vi "IMU model SUBVI.vi"(11 "Enum 3":enum16{"None", "Disc", "Box", "STL"}(ring)=enum."Disc") -> (3 "SceneObject out":refnum<vi>)   [LabVIEW 2021, in "IMU Display.lvlib"]
uses:
  <vilib>/picture/3D Picture Control/Object/Create Object (name).vi
  <vilib>/picture/3D Picture Control/Object/Create Object (drawable).vi
  <vilib>/picture/3D Picture Control/Object/Add Object (no reference).vi
  IMU Display.lvlib
  <vilib>/picture/3D Picture Control/NI_3D Picture Control.lvlib
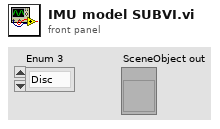
[diagram p1: front panel]
types:
  T1 = cluster{"Red":sgl, "Green":sgl, "Blue":sgl, "Alpha":sgl}
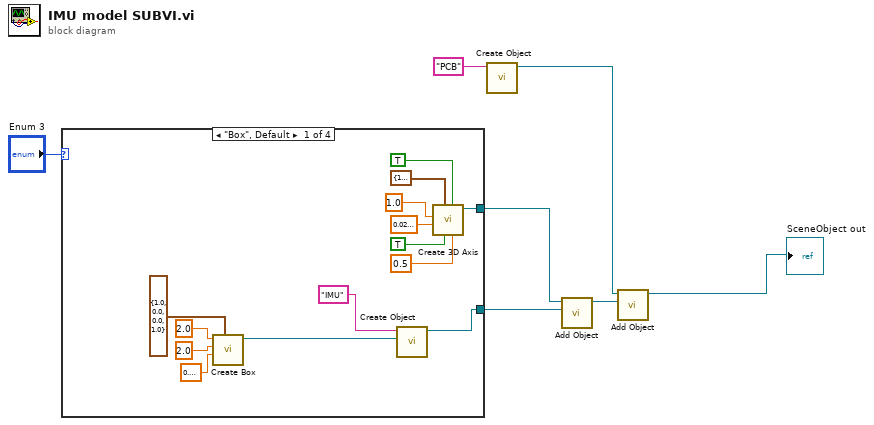
[diagram p0: block diagram]
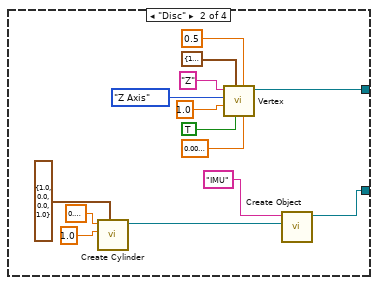
[diagram p2: hidden frame]
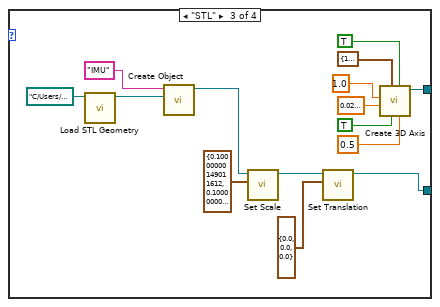
[diagram p3: hidden frame]
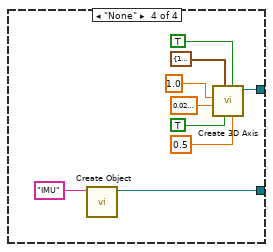
[diagram p4: hidden frame]
diagram:
  n1 = case shown="\"Box\", Default" "Enum 3" {
    tunnel: [w16 w32 w43 w58] -> w2
    tunnel: [w8 w23 w36 w51] -> w4
    frame "Box", Default {
      n2 = call <vilib>:"Create Box.vi"("Color"=T1 {"Red"=1.0, "Green"=0.0, "Blue"=0.0, "Alpha"=1.0}, "Length Z"=sgl 0.2, "Length Y"=sgl 2.0, "Length X"=sgl 2.0) -> ("New Box Refnum"=w17:refnum<vi>)  [unwired: 6 in, 1 out]
      n3 = call-poly <vilib>:"Create Object.vi"("Geometry"=w17, "Name"="IMU") -> ("Scene:New Object"=w16:refnum<vi>)  [unwired: 8 in, 1 out]
      n4 = call <vilib>:"Create 3D Axis.vi"("Character Size"=sgl 0.5, "Half plane?"=TRUE, "Axis label?"=TRUE, "Color"=T1 {"Red"=1.0, "Green"=0.0, "Blue"=0.0, "Alpha"=1.0}, "Radius"=sgl 0.03, "Length"=sgl 1.0) -> ("New Object Refnum"=w8:refnum<vi>)  [unwired: 4 in, 1 out]
    }
    frame "Disc" {
      n5 = call <vilib>:"Create Cylinder.vi"("Color"=T1 {"Red"=1.0, "Green"=0.0, "Blue"=0.0, "Alpha"=1.0}, "Radius"=sgl 1.0 ("Length Y"), "Height"=sgl 0.2 ("Length Z")) -> ("New Cylinder Refnum"=w33:refnum<vi>)  [unwired: 7 in, 1 out]
      n6 = call "Vertex.vi"("Radius"=sgl 0.01, "Font Size"=sgl 0.5 ("Character Size"), "Vertex label?"=TRUE ("Axis label?"), "Color"=T1 {"Red"=1.0, "Green"=0.0, "Blue"=0.0, "Alpha"=1.0}, "Length"=sgl 1.0, "Enum"=enum16{"X Axis", "Y Axis", "Z Axis"}."Z Axis", "Name"="Z") -> ("New Object Refnum"=w23:refnum<vi>)  [unwired: 3 in, 1 out]
      n7 = call-poly <vilib>:"Create Object.vi"("Geometry"=w33, "Name"="IMU") -> ("Scene:New Object"=w32:refnum<vi>)  [unwired: 8 in, 1 out]
    }
    frame "STL" {
      n8 = call <vilib>:"Load STL Geometry.vi"("Model File"=path "C:/Users/gigi3/OneDrive - KU Leuven/Thesis/Labview/sparkfun-9dof-imu-breakout-icm-20948-qwiic-1.snapshot.3/SparkFun_IMU_Breakout_ICM-20948 v4 v1.stl") -> ("New Mesh Refnum"=w49:refnum<vi>)  [unwired: 9 in, 1 out]
      n9 = call-poly <vilib>:"Create Object.vi"("Geometry"=w49, "Name"="IMU") -> ("Scene:New Object"=w44:refnum<vi>)  [unwired: 8 in, 1 out]
      n10 = call <vilib>:"Set Scale.vi"("Scale"=cluster{"X":sgl, "Y":sgl, "Z":sgl} {"X"=0.1, "Y"=0.1, "Z"=0.09999999}, "Scene Object"=w44) -> ("Scaled Object"=w46:refnum<vi>)  [unwired: 8 in, 1 out]
      n11 = call <vilib>:"Set Translation.vi"("Translation"=cluster{"X":sgl, "Y":sgl, "Z":sgl} {"X"=0.0, "Y"=0.0, "Z"=0.0}, "Scene Object"=w46) -> ("Translated Object"=w43:refnum<vi>)  [unwired: 8 in, 1 out]
      n12 = call <vilib>:"Create 3D Axis.vi"("Character Size"=sgl 0.5, "Half plane?"=TRUE, "Axis label?"=TRUE, "Color"=T1 {"Red"=1.0, "Green"=0.0, "Blue"=0.0, "Alpha"=1.0}, "Radius"=sgl 0.03, "Length"=sgl 1.0) -> ("New Object Refnum"=w36:refnum<vi>)  [unwired: 4 in, 1 out]
    }
    frame "None" {
      n13 = call-poly <vilib>:"Create Object.vi"("Name"="IMU") -> ("Scene:New Object"=w58:refnum<vi>)  [unwired: 9 in, 1 out]
      n14 = call <vilib>:"Create 3D Axis.vi"("Character Size"=sgl 0.5, "Half plane?"=TRUE, "Axis label?"=TRUE, "Color"=T1 {"Red"=1.0, "Green"=0.0, "Blue"=0.0, "Alpha"=1.0}, "Radius"=sgl 0.03, "Length"=sgl 1.0) -> ("New Object Refnum"=w51:refnum<vi>)  [unwired: 4 in, 1 out]
    }
  }
  n15 = call-poly <vilib>:"Create Object.vi"("Name"="PCB") -> ("Scene:New Object"=w7:refnum<vi>)  [unwired: 9 in, 1 out]
  n16 = call-poly <vilib>:"Add Object.vi"("New Object In"=w2, "Scene Object In"=w4) -> ("Scene Object Out"=w6:refnum<vi>)  [unwired: 8 in, 1 out]
  n17 = call-poly <vilib>:"Add Object.vi"("New Object In"=w6, "Scene Object In"=w7) -> ("Scene Object Out"=→"SceneObject out":refnum<vi>)  [unwired: 8 in, 1 out]
